vi "Log Data.vi"(8 "error in (no error)":errorcluster, 10 "Data Queue":refnum<queue>, 11 "Logging Configuration":T1) -> (0 "error out":errorcluster)   [LabVIEW 2014, in "Demonstrator Logging.lvlib"]
doc: "This VI uses the TDMS Write function to write data to a TDMS file."
uses:
  Demonstrator Logging.lvlib
  Logging Configuration.ctl
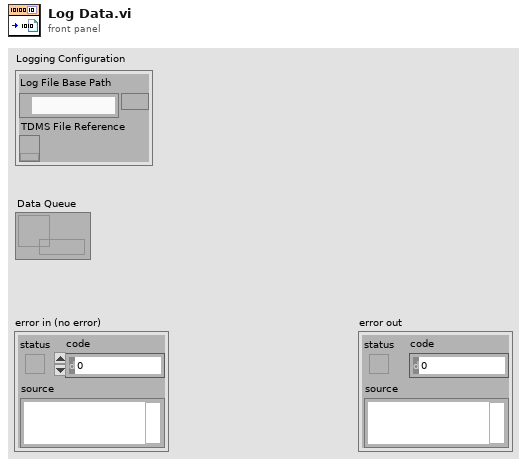
[diagram p1: front panel]
types:
  T1 = typedef "Demonstrator Logging.lvlib/Logging Configuration.ctl" = cluster{"Log File Base Path":path, "TDMS File Reference":refnum<k34>}
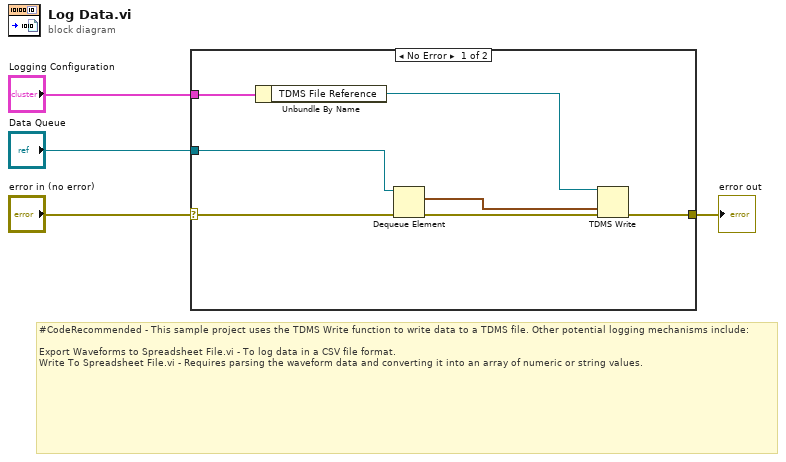
[diagram p0: block diagram]
diagram:
  # "#CodeRecommended - This sample project uses the TDMS Write function to write data to a TDMS file. Other potential logging mechanisms include:\n\nExport Waveforms to Spreadsheet File.vi - To log data in a CSV file format.\nWrite To Spreadsheet File.vi - Requires parsing the waveform data and converting it into an array of numeric or string values."
  n1 = case shown="No Error" "error in (no error)" {
    selector: "error in (no error)" -> [w9 w12]
    tunnel: "Logging Configuration" -> [w11 _]
    tunnel: "Data Queue" -> [w8 _]
    tunnel: [w10 w12] -> w2
    frame No Error {
      n2 = Unbundle By Name(w11) -> ("TDMS File Reference"=w5:refnum<k34>)
      n3 = Dequeue Element(queue=w8, error in (no error)=w9) -> (element=w6:waveform(dbl)[], error out=w7:errorcluster)  [unwired: 1 in, 2 out]
      n4 = TDMS Write(0:w5, 9:w6, 11:w7) -> (15:w10:errorcluster)  [unwired: 3 in, 3 out]
    }
    frame Error {
    }
  }
  "error out" <- w2
